vi "Read Tick Colors.vi"(9 "Scale in":refnum<class "Scale.lvclass">) -> (3 "Scale out":refnum<class "Scale.lvclass">, 4 "Tick Colors":T1)   [LabVIEW 2014, in "Raspberry Pi Compatible Compiler for LabVIEW.lvlib" / "Scale.lvclass"]
uses:
  Scale.lvclass
  <vilib>/Utility/miscctls.llb/LVTickColorsTypeDef.ctl
  Scale.lvclass/Scale.ctl
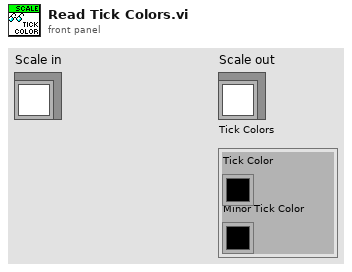
[diagram p1: front panel]
types:
  T1 = typedef "LVTickColorsTypeDef.ctl" = cluster{"Tick Color":u32, "Minor Tick Color":u32}
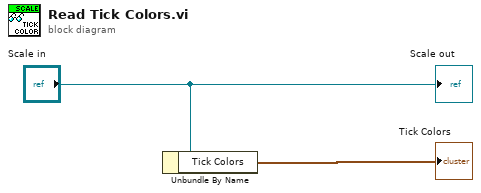
[diagram p0: block diagram]
diagram:
  n1 = Unbundle By Name("Scale in") -> ("Tick Colors"=→"Tick Colors":T1)
  "Scale out" <- "Scale in"
